vi "gui_T1_analysis.vi"(6 "fitted_signal":T3, 8 "fit_parameters":T4, 9 "T1 curve":cluster{dbl[], "dark_time_us":dbl[]}, 10 "T1_parameters":T2, 11 "timetags":u32[][](array[numeric])) -> ()   [LabVIEW 2014]
panel:
  in  "save_file":bool
  out "delta":dbl format="%#_3f"
  in  "show_photons":bool
  in  "show_flags":bool
  out "read_width-ph_1":T1(graph)
  in  "use_proposed":bool
  out "proposed_read_width_us":dbl
  out "proposed_correction_us":dbl
  out "histogram":cluster{"histogram":i32[], "q_photons":i32[]}(graph)
  out "file_name":string caption="File"
  out "sampling_mode":enum16{"Normal", "Sweep"}(ring)
  out "quality":bool
  out "mse":dbl caption="Mean Square Error" format="%#.2e"
  out "T1_us":dbl format="%#.3g"
  out "T1 curves":cluster{dbl[], "dark_time_us":dbl[]}[](graph)
  in  "correction_us":dbl caption="Delay"
  out "stop_count_photon":u32(colorbox)=16776704 caption="Stop Count & photon"
  out "stop_count":u32(colorbox)=6618880 caption="Stop Count"
  out "start_count_photon":u32(colorbox)=14417925 caption="Start Count & photon"
  out "start_count":u32(colorbox)=255 caption="Start Count"
  out "photon":u32(colorbox)=16448250 caption="Photon"
  out "noPhoton":u32(colorbox) caption="No Photon"
  out "photons_chart":u32[][](graph)
  in  "load_file":bool
  in  "refit":bool
  in  "read_width_us":dbl=0.3 caption="Width" min=0.0 max=10000.0 format="%#.3f"
  out "read_delay_us":dbl caption="Delay"
  out "min_step":dbl format="%#.3f"
  out "q_samples":i32=100
  out "dt_stop_us":dbl=1.0
  out "dt_start_us":dbl=0.1
  in  "stop":bool
  out "repetitions":i32=100 caption="Repetitions" min=1 step=1
  out "pulse_width_us":dbl=3.0 caption="Pulse width"
  # "Dark time [us]"
  # "*"
  # "*"
  # "us"
  # "*read_width_us and correction_us have to be multiple of 10ns\n*** start and stop markers are inside the detection gate. [start, stop]"
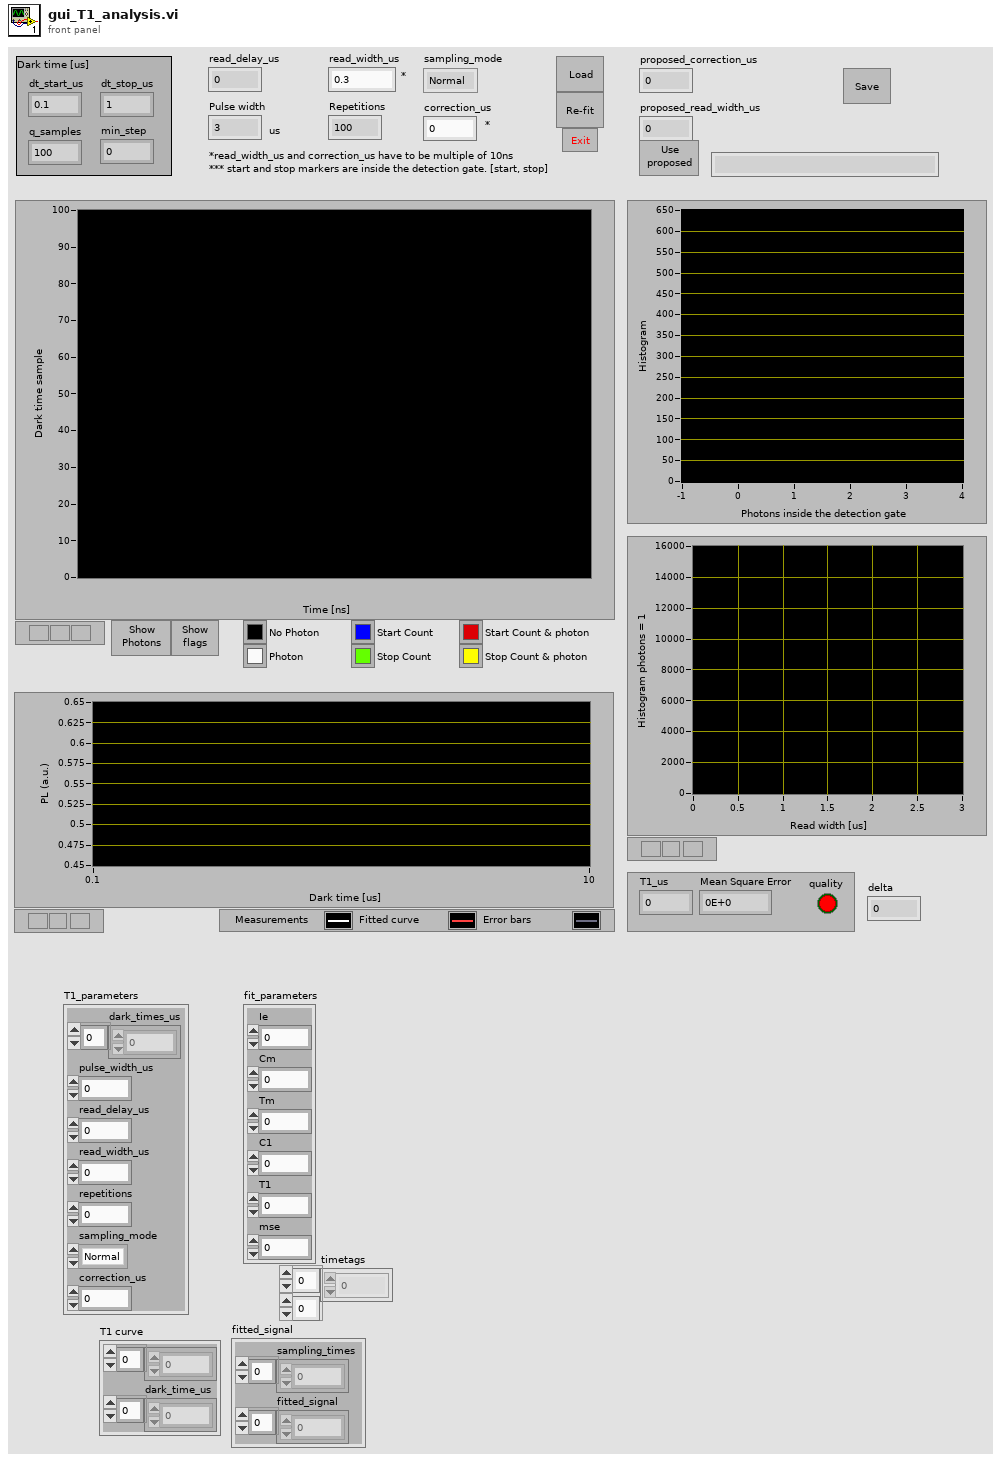
[diagram p1: front panel]
types:
  T1 = cluster{"read_widths_us":dbl[], "histogram_q1":i32[]}
  T2 = cluster{"dark_times_us":dbl[], "pulse_width_us":dbl, "read_delay_us":dbl, "read_width_us":dbl, "repetitions":i32, "sampling_mode":enum16{"Normal", "Sweep"}, "correction_us":dbl}
  T3 = cluster{"sampling_times":dbl[], "fitted_signal":dbl[]}
  T4 = cluster{"Ie":dbl, "Cm":dbl, "Tm":dbl, "C1":dbl, "T1":dbl, "mse":dbl}
  T5 = enum16{"standby", "doT1", "abort", "save", "re-fit", "load"}
  T6 = enum16{"standby", "doT1", "abort", "save", "re-fit", "load", "refresh"}
  T7 = enum16{"standby", "doT1", "abort", "save", "re-fit", "load", "refresh", "use_proposed"}
  T8 = cluster{"dark_times_us":dbl[], "fitted_signal":dbl[]}[]
  T9 = cluster{"dark_times":dbl[], "fitted_signal":dbl[]}
  T10 = cluster{"dark_times_us":dbl[], "measured_signal":dbl[]}
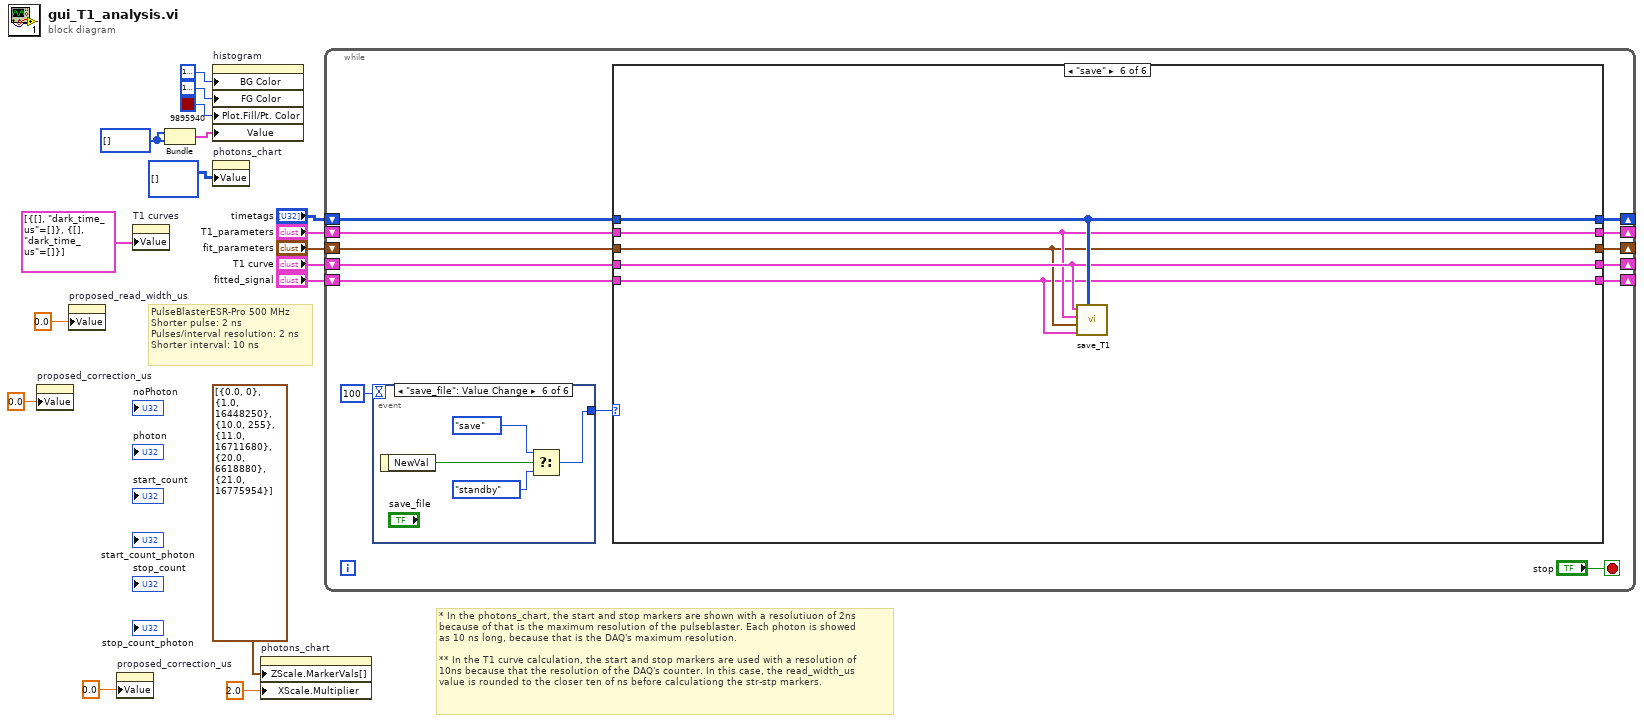
[diagram p0: block diagram]
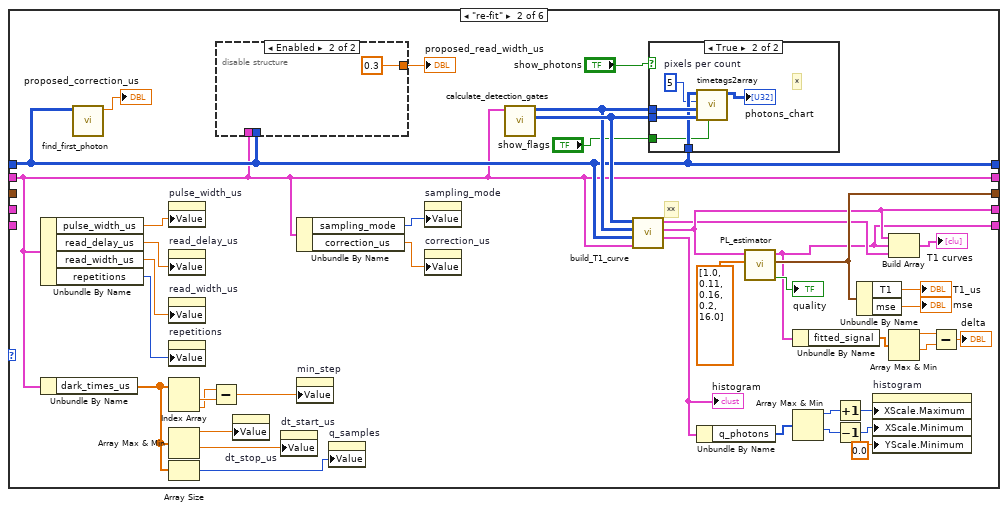
[diagram p3: hidden frame]
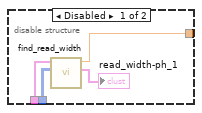
[diagram p5: hidden frame]
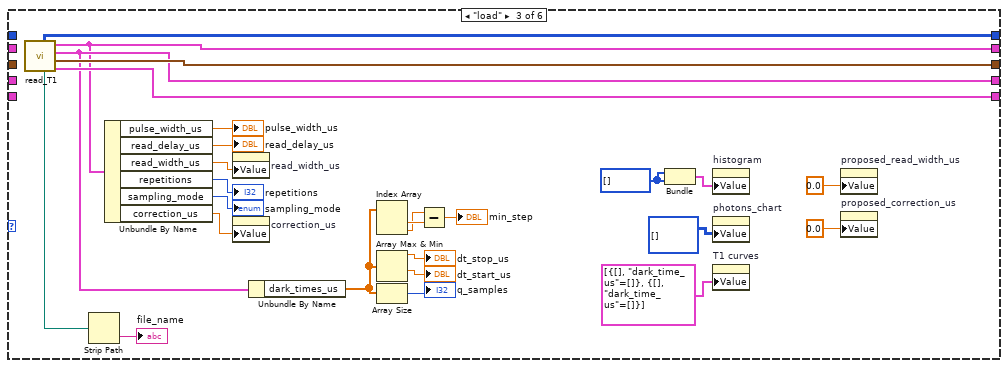
[diagram p6: hidden frame]
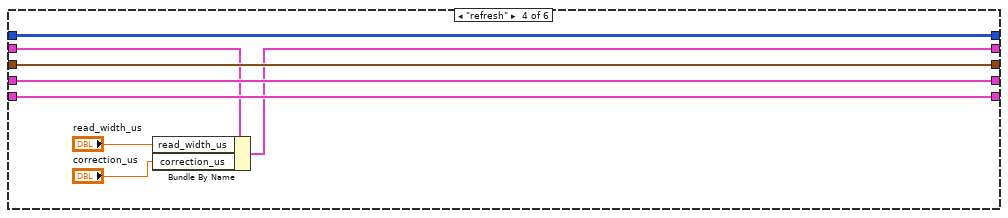
[diagram p7: hidden frame]
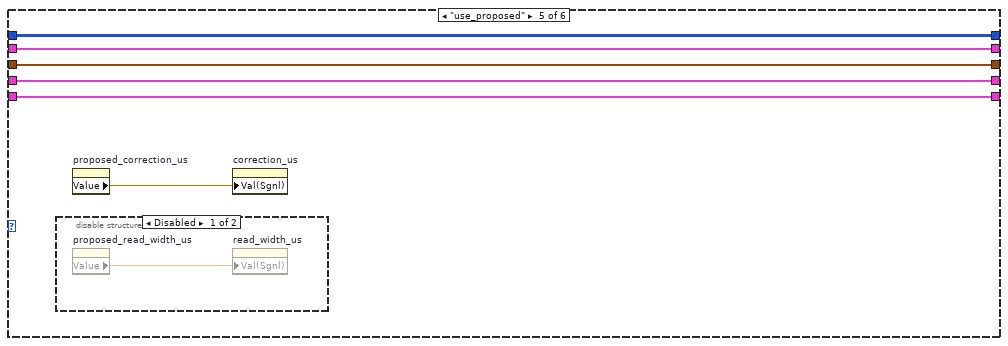
[diagram p8: hidden frame]
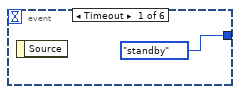
[diagram p10: hidden frame]
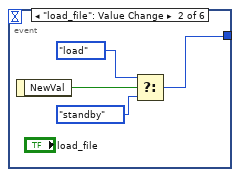
[diagram p11: hidden frame]
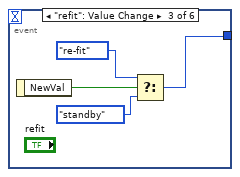
[diagram p12: hidden frame]
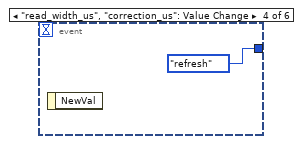
[diagram p13: hidden frame]
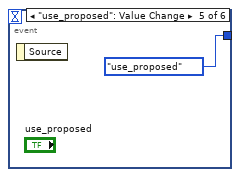
[diagram p14: hidden frame]
diagram:
  w6 = i32[] []
  # "* In the photons_chart, the start and stop markers are shown with a resolutiuon of 2ns \nbecause of that is the maximum resolution of the pulseblaster. Each photon is showed\nas 10 ns long, because that is the DAQ's maximum resolution.\n\n** In the T1 curve calculation, the start and stop markers are used with a resolution of\n10ns because that the resolution of the DAQ's counter. In this case, the read_width_us\nvalue is rounded to the closer ten of ns before calculationg the str-stp markers."
  # "PulseBlasterESR-Pro 500 MHz \nShorter pulse: 2 ns\nPulses/interval resolution: 2 ns\nShorter interval: 10 ns"
  n1 = property on="proposed_correction_us" class="DigNum (strict)"("Value"=0.0 ("proposed_correction_us")) -> ()  [unwired: 2 in, 2 out]
  n2 = property on="proposed_read_width_us" class="DigNum (strict)"("Value"=0.0 ("proposed_read_width_us")) -> ()  [unwired: 2 in, 2 out]
  n3 = property on="proposed_correction_us" class="DigNum (strict)"("Value"=0.0 ("proposed_correction_us")) -> ()  [unwired: 2 in, 2 out]
  n4 = property on="T1 curves" class="XYGraph (strict)"("Value"=cluster{dbl[], "dark_time_us":dbl[]}[] [{[], "dark_time_us"=[]}, {[], "dark_time_us"=[]}] ("T1 curves")) -> ()  [unwired: 2 in, 2 out]
  n5 = Bundle(w6, w6) -> (w5:cluster{i32[], i32[]})  [unwired: 1 in]
  n6 = property on="histogram" class="XYGraph (strict)"("BG Color"=u32 16777222 ("Plot Area:Colors:FG Color"), "FG Color"=u32 16777228 ("Plot Area:Colors:FG Color"), "Plot.Fill/Pt. Color"=u32 9895940 ("Plot Area:Colors:FG Color"), "Value"=w5) -> ()  [unwired: 2 in, 2 out]
  n7 = property on="photons_chart" class="IntGraph (strict)"("Value"=i32[][] []) -> ()  [unwired: 2 in, 2 out]
  n8 = property on="photons_chart" class="IntGraph (strict)"("ZScale.MarkerVals[]"=cluster{dbl, u32}[] [{0.0, 0}, {1.0, 16448250}, {10.0, 255}, {11.0, 16711680}, {20.0, 6618880}, {21.0, 16775954}] ("Z Scale.Marker Values[]"), "XScale.Multiplier"=2.0 ("X Scale.Offset and Multiplier:Multiplier")) -> ()  [unwired: 2 in, 2 out]
  n9 = while {
    shift-right: [w20] -> _
    shift-left: "T1_parameters" -> [w27]
    shift-right: [w19] -> _
    shift-left: "fit_parameters" -> [w26]
    shift-right: [w18] -> _
    shift-left: "T1 curve" -> [w25]
    shift-right: [w24] -> _
    shift-left: "fitted_signal" -> [w23]
    shift-right: [w21] -> _
    shift-left: "timetags" -> [w22]
    stop <- "stop" stop-if-true
    n10 = event shown="[5] \"save_file\": Value Change" {
      selector: _ -> [_ _ _ _ _ _]
      dyn-events: _ -> [_ _ _ _ _ _]
      timeout: 100 -> [_ _ _ _ _ _]
      tunnel: [T5."standby" w136 w141 T6."refresh" T7."use_proposed" w145] -> w28
      event Timeout {
        n11 = event-data() -> ()  [unwired: 1 in, 1 out]
      }
      event "load_file": Value Change {
        n12 = event-data() -> ("NewVal"=w137:bool)  [unwired: 1 in]
        n13 = Select(t=T5."load", s=w137, f=T5."standby") -> (s? t:f=w136:T5)
      }
      event "refit": Value Change {
        n14 = event-data() -> ("NewVal"=w142:bool)  [unwired: 1 in]
        n15 = Select(t=T5."re-fit", s=w142, f=T5."standby") -> (s? t:f=w141:T5)
      }
      event "read_width_us", "correction_us": Value Change {
        n16 = event-data() -> ()  [unwired: 1 in, 1 out]
      }
      event "use_proposed": Value Change {
        n17 = event-data() -> ()  [unwired: 1 in, 1 out]
      }
      event "save_file": Value Change {
        n18 = event-data() -> ("NewVal"=w146:bool)  [unwired: 1 in]
        n19 = Select(t=T5."save", s=w146, f=T5."standby") -> (s? t:f=w145:T5)
      }
    }
    n20 = case shown="\"save\"" w28 {
      tunnel: w27 -> [w35 w45 _ w117 w125 w131]
      tunnel: w26 -> [w34 _ _ w120 w124 w130]
      tunnel: w25 -> [w33 _ _ w119 w123 w132]
      tunnel: [w32 w40 w113 w118 w122 w129] -> w24
      tunnel: w23 -> [w32 _ _ w118 w122 w129]
      tunnel: [w31 w46 w96 w121 w126 w133] -> w21
      tunnel: w22 -> [w31 w46 _ w121 w126 w133]
      tunnel: [w35 w45 w99 w116 w125 w131] -> w20
      tunnel: [w34 w75 w112 w120 w124 w130] -> w19
      tunnel: [w33 w44 w108 w119 w123 w132] -> w18
      frame "standby", Default {
      }
      frame "re-fit" {
        # "**"
        n21 = Unbundle By Name(w45) -> ("pulse_width_us"=w65:dbl, "read_delay_us"=w64:dbl, "read_width_us"=w63:dbl, "repetitions"=w62:i32)
        n22 = Unbundle By Name(w45) -> ("dark_times_us"=w70:dbl[])
        n23 = call "find_first_photon.vi"("timetags"=w46) -> ("Numeric"=→"proposed_correction_us":dbl)  [unwired: 10 in]
        n24 = property on="pulse_width_us" class="DigNum (strict)"("Value"=w65) -> ()  [unwired: 2 in, 2 out]
        n25 = property on="read_delay_us" class="DigNum (strict)"("Value"=w64) -> ()  [unwired: 2 in, 2 out]
        n26 = property on="read_width_us" class="DigNum (strict)"("Value"=w63) -> ()  [unwired: 2 in, 2 out]
        n27 = property on="repetitions" class="DigNum (strict)"("Value"=w62) -> ()  [unwired: 2 in, 2 out]
        n28 = Index Array(array=w70) -> (element #1=w72:dbl, element #2=w71:dbl)  [unwired: 2 in]
        n29 = Array Max & Min(array=w70) -> (max value=w69:dbl, min value=w68:dbl)  [unwired: 2 out]
        n30 = Array Size(array=w70) -> (size(s)=w67:i32)
        n31 = Subtract(x=w71, y=w72) -> (x-y=w66:dbl)
        n32 = disable-structure shown="Enabled" {
          disable-tunnel: [w86 0.3 ("proposed_read_width_us")] -> w48
          disable-tunnel: w46 -> [w85 _]
          disable-tunnel: w45 -> [w84 _]
          frame Disabled {
            n33 = call "find_read_width.vi"("timetags"=w85, "T1_parameters"=w84) -> ("hist_q1-read_width"=→"read_width-ph_1":T1, "proposed_read_width_us"=w86:dbl)  [unwired: 8 in]
          }
          frame Enabled {
          }
        }
        "proposed_read_width_us" <- w48
        n34 = property on="dt_stop_us" class="DigNum (strict)"("Value"=w69) -> ()  [unwired: 2 in, 2 out]
        n35 = property on="dt_start_us" class="DigNum (strict)"("Value"=w68) -> ()  [unwired: 2 in, 2 out]
        n36 = Unbundle By Name(w45) -> ("sampling_mode"=w57:enum16{"Normal", "Sweep"}, "correction_us"=w56:dbl)
        n37 = property on="min_step" class="DigNum (strict)"("Value"=w66) -> ()  [unwired: 2 in, 2 out]
        n38 = property on="q_samples" class="DigNum (strict)"("Value"=w67) -> ()  [unwired: 2 in, 2 out]
        n39 = property on="sampling_mode" class="Enum (strict)"("Value"=w57) -> ()  [unwired: 2 in, 2 out]
        n40 = property on="correction_us" class="DigNum (strict)"("Value"=w56) -> ()  [unwired: 2 in, 2 out]
        n41 = call "calculate_detection_gates.vi"("T1_parameters"=w45) -> ("start_read"=w59:u32[][], "stop_read"=w58:u32[][])  [unwired: 9 in]
        n42 = call "build_T1_curve.vi"("T1_parameters"=w45, "timetags"=w46, "stop_read"=w58, "start_read"=w59) -> ("histogram"=w55:cluster{"q_photons":i32[], "histogram":i32[]}, "T1 curve"=w44:cluster{dbl[], "dark_time_us":dbl[]}, "error_bars"=w43:cluster{"dark_times_us":dbl[], dbl[]})  [unwired: 5 in]
        "histogram" <- w55
        n43 = case shown="True" "show_photons" {
          tunnel: w59 -> [_ w81]
          tunnel: w58 -> [_ w80]
          tunnel: w46 -> [_ w79]
          tunnel: "show_flags" -> [_ w78]
          frame False {
          }
          frame True {
            w77 = u32 5  # pixels per count
            # "*"
            n44 = call "timetags2array.vi"("show_flags"=w78, "start_read"=w81, "stop_read"=w80, "pixels/count"=w77, "timetags"=w79) -> ("photons_chart"=→"photons_chart":u32[][])  [unwired: 6 in]
          }
        }
        n45 = Unbundle By Name(w55) -> ("q_photons"=w54:i32[])
        n46 = call "PL_estimator.vi"("initial parameters"=dbl[] [1.0, 0.11, 0.16, 0.2, 16.0], "measured_signal"=w44) -> ("quality_check"=→"quality":bool, "fit_parameters"=w75:T4, "fitted_signal"=w40:T3)  [unwired: 7 in]
        n47 = Unbundle By Name(w40) -> ("fitted_signal"=w39:dbl[])
        n48 = Array Max & Min(array=w54) -> (max value=w53:i32, min value=w51:i32)  [unwired: 2 out]
        n49 = Increment(x=w53) -> (x+1=w52:i32)
        n50 = Decrement(x=w51) -> (x-1=w50:i32)
        n51 = Unbundle By Name(w75) -> ("T1"=→"T1_us":dbl, "mse"=→"mse":dbl)
        n52 = property on="histogram" class="XYGraph (strict)"("XScale.Maximum"=w52, "XScale.Minimum"=w50, "YScale.Minimum"=0.0 ("Y Scale.Range:Minimum")) -> ()  [unwired: 2 in, 2 out]
        n53 = Build Array(w44, w40, w43) -> (→"T1 curves":T8)
        n54 = Array Max & Min(array=w39) -> (max value=w38:dbl, min value=w37:dbl)  [unwired: 2 out]
        n55 = Subtract(x=w38, y=w37) -> (x-y=→"delta":dbl)
      }
      frame "load" {
        w93 = i32[] []
        n56 = call "read_T1.vi"() -> ("fitted_signal"=w113:T9, "fit_parameters"=w112:T4, "T1_curve"=w108:T10, "T1_parameters"=w99:T2, "file_path"=w95:path, "timetags"=w96:u32[][])  [unwired: 6 in]
        n57 = Strip Path(path=w95) -> (name=→"file_name":string)  [unwired: 1 out]
        n58 = Unbundle By Name(w99) -> ("pulse_width_us"=→"pulse_width_us":dbl, "read_delay_us"=→"read_delay_us":dbl, "read_width_us"=w100:dbl, "repetitions"=→"repetitions":i32, "sampling_mode"=→"sampling_mode":enum16{"Normal", "Sweep"}, "correction_us"=w97:dbl)
        n59 = property on="read_width_us" class="DigNum (strict)"("Value"=w100) -> ()  [unwired: 2 in, 2 out]
        n60 = property on="correction_us" class="DigNum (strict)"("Value"=w97) -> ()  [unwired: 2 in, 2 out]
        n61 = Unbundle By Name(w108) -> ("dark_times_us"=w104:dbl[])
        n62 = Index Array(array=w104) -> (element #1=w103:dbl, element #2=w102:dbl)  [unwired: 2 in]
        n63 = Array Max & Min(array=w104) -> (max value=→"dt_stop_us":dbl, min value=→"dt_start_us":dbl)  [unwired: 2 out]
        n64 = Array Size(array=w104) -> (size(s)=→"q_samples":i32)
        n65 = Subtract(x=w102, y=w103) -> (x-y=→"min_step":dbl)
        n66 = Bundle(w93, w93) -> (w92:cluster{i32[], i32[]})  [unwired: 1 in]
        n67 = property on="histogram" class="XYGraph (strict)"("Value"=w92) -> ()  [unwired: 2 in, 2 out]
        n68 = property on="photons_chart" class="IntGraph (strict)"("Value"=i32[][] []) -> ()  [unwired: 2 in, 2 out]
        n69 = property on="T1 curves" class="XYGraph (strict)"("Value"=cluster{dbl[], "dark_time_us":dbl[]}[] [{[], "dark_time_us"=[]}, {[], "dark_time_us"=[]}] ("T1 curves")) -> ()  [unwired: 2 in, 2 out]
        n70 = property on="proposed_read_width_us" class="DigNum (strict)"("Value"=0.0 ("proposed_read_width_us")) -> ()  [unwired: 2 in, 2 out]
        n71 = property on="proposed_correction_us" class="DigNum (strict)"("Value"=0.0 ("proposed_correction_us")) -> ()  [unwired: 2 in, 2 out]
      }
      frame "refresh" {
        n72 = Bundle By Name(cluster=w117, "read_width_us"="read_width_us", "correction_us"="correction_us") -> (w116:T2)
      }
      frame "use_proposed" {
        n73 = disable-structure shown="Disabled" {
          frame Disabled {
            n74 = property on="proposed_read_width_us" class="DigNum (strict)"() -> ("Value"=w128:dbl)  [unwired: 2 in, 2 out]
            n75 = property on="read_width_us" class="DigNum (strict)"("Val(Sgnl)"=w128) -> ()  [unwired: 2 in, 2 out]
          }
          frame Enabled {
          }
        }
        n76 = property on="proposed_correction_us" class="DigNum (strict)"() -> ("Value"=w127:dbl)  [unwired: 2 in, 2 out]
        n77 = property on="correction_us" class="DigNum (strict)"("Val(Sgnl)"=w127) -> ()  [unwired: 2 in, 2 out]
      }
      frame "save" {
        n78 = call "save_T1.vi"("T1_curve_in"=w132, "timetags"=w133, "T1_parameters"=w131, "fit_parameters"=w130, "fitted_signal_in"=w129) -> ()  [unwired: 4 in]
      }
    }
  }
